vi "LoadControlPanel.vi"(8 "error in (no error)":errorcluster, 10 "Actor In":refnum<class "Actor.lvclass">, 11 "DataLogger in":refnum<class "DataLogger.lvclass">) -> (0 "error out":errorcluster, 3 "DataLogger out":refnum<class "DataLogger.lvclass">)   [LabVIEW 2020, in "DataLogger.lvlib" / "DataLogger.lvclass"]
uses:
  DataLogger.lvclass
  DataLoggerUI/DataLoggerUI.lvclass
  Hardware Abstraction Layer/Component/Device/Device/DataExchange.ctl
  Interface/DataListener/DataListener.lvclass
  Hardware Abstraction Layer/Component/GenericActor/GenericActor/GenericController.lvclass
  C:/Program Files/National Instruments/LabVIEW 2020/vi.lib/ActorFramework/Actor/Actor.lvclass
  <vilib>/ActorFramework/Actor/Actor.lvclass
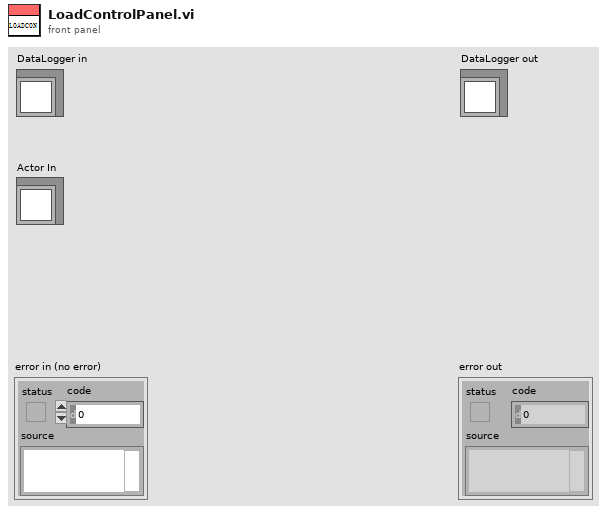
[diagram p1: front panel]
types:
  T1 = typedef "DataListener.lvclass/DataExchange.ctl" = cluster{"Source":string, "Destination":string, "Description":string, "value":variant}
  T2 = cluster{"StreamToDisk?":bool, "SingleStack?":bool, "Alert when finish?":bool, "TiffFileFullPath":path, "StreamFileFullPath":path}
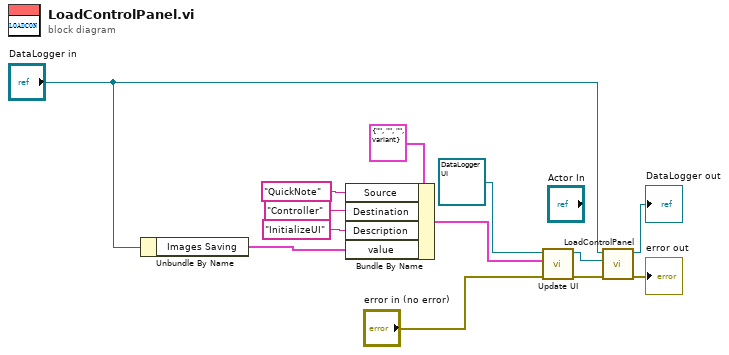
[diagram p0: block diagram]
diagram:
  n1 = Unbundle By Name("DataLogger in") -> ("Images Saving"=w1:T2)
  n2 = Bundle By Name(cluster=T1 {"Source"="", "Destination"="", "Description"="", "value"=variant} ("DataExchange"), "Source"="QuickNote", "Destination"="Controller", "Description"="InitializeUI", "value"=w1) -> (w3:T1)
  n3 = call-dynamic "Update UI.vi"("error in (no error)"="error in (no error)", "DataExchange"=w3, "Controller Template in"=refnum<class "DataLoggerUI.lvclass"> refnum ("DataLogger.lvlib:DataLoggerUI.lvclass")) -> ("error out"=w10:errorcluster, "Controller Template out"=w8:refnum<class "DataLoggerUI.lvclass">)  [unwired: 7 in]
  n4 = call-parent "LoadControlPanel.vi"("error in (no error)"=w10, "Actor In"=w8, "GRMActor in"="DataLogger in") -> ("error out"=→"error out":errorcluster, "GRMActor out"=→"DataLogger out":refnum<class "DataLogger.lvclass">)  [unwired: 7 in]
